vi "DataToGenerateVar.vi"(6 "Header":string[](array[string]), 8 "error in (no error)":errorcluster, 10 "Data in":string[][](array[string]), 11 "Variant":variant) -> (0 "error out":errorcluster, 3 "Data":variant[](array[variant]))   [LabVIEW 2014, in "TableLogger_Actor.lvlib" / "TableLogger_Actor.lvclass"]
uses:
  TableLogger_Actor.lvclass
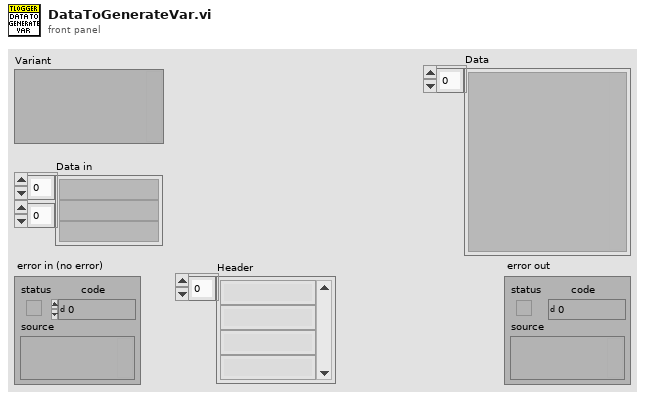
[diagram p1: front panel]
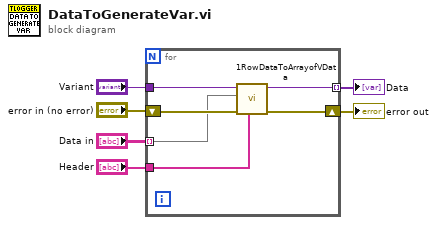
[diagram p0: block diagram]
diagram:
  n1 = for {
    tunnel: [w12] -> w3 mode=indexing
    shift-right: [w10] -> w6
    shift-left: "error in (no error)" -> [w11]
    tunnel: "Data in" -> [w8] mode=indexing
    tunnel: "Variant" -> [w9]
    tunnel: "Header" -> [w7]
    n2 = call "1RowDataToArrayofVData.vi"("Header"=w7, "error in (no error)"=w11, "Data in"=w8, "Variant"=w9) -> ("error out"=w10:errorcluster, "Varaint Out"=w12:variant)  [unwired: 6 in]
  }
  "error out" <- w6
  "Data" <- w3
